vi "Set Velocity Setpoint.vi"(8 "error in (no error)":errorcluster, 10 "ccw velocity (rpm)":dbl, 11 "KUKA youBot gripper motor in":refnum<class "NI_Robotics_KUKA youBot Gripper Motor_EtherCAT.lvclass">) -> (0 "error out":errorcluster, 3 "KUKA youBot gripper motor out":refnum<class "NI_Robotics_KUKA youBot Gripper Motor_EtherCAT.lvclass">)   [LabVIEW 2017, in "NI_Robotics_KUKA youBot Host.lvlib" / "NI_Robotics_KUKA youBot Gripper Motor_EtherCAT.lvclass"]
uses:
  <vilib>/robotics/KUKA youBot/Motor/Gripper Motor EtherCAT/NI_Robotics_KUKA youBot Gripper Motor_EtherCAT.lvclass
  <vilib>/robotics/KUKA youBot/Motor/Gripper Motor EtherCAT/NI_Robotics_KUKA youBot Gripper Motor_EtherCAT.lvclass/NI_Robotics_KUKA youBot Gripper Motor_EtherCAT.ctl
  <vilib>/robotics/KUKA youBot/EtherCAT/EtherCAT Command.ctl
  <vilib>/robotics/KUKA youBot/EtherCAT/CmdCtrls/Param Cmd.ctl
  <vilib>/robotics/KUKA youBot/NI_Robotics_KUKA youBot Host.lvlib
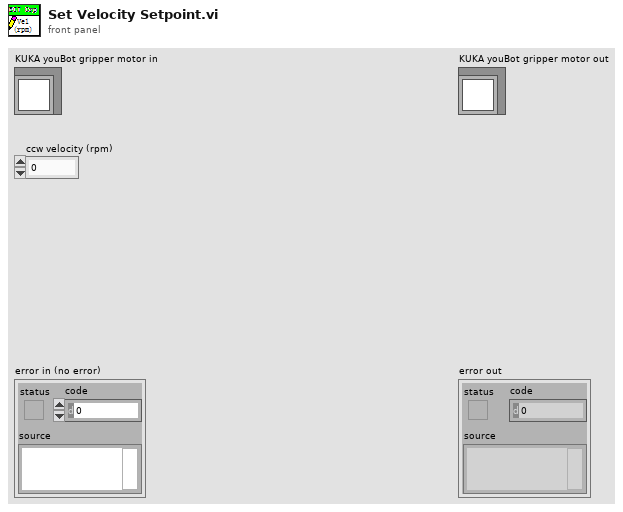
[diagram p1: front panel]
types:
  T1 = typedef "NI_Robotics_KUKA youBot Host.lvlib/EtherCAT Command.ctl" = cluster{"Module":u8, "Cmd":T2, "Type":u8, "Bank":u8, "Val":u32}
  T2 = typedef "NI_Robotics_KUKA youBot Host.lvlib/Param Cmd.ctl" = u8
  T3 = typedef "NI_Robotics_KUKA youBot Host.lvlib/Mater Handler.ctl" = i32
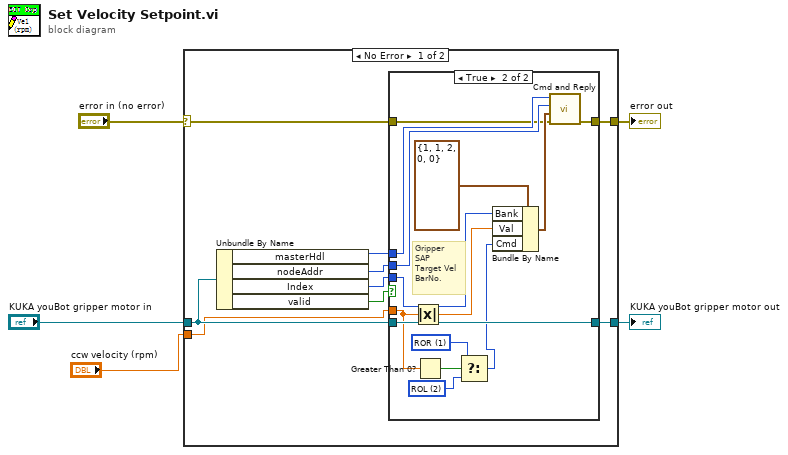
[diagram p0: block diagram]
diagram:
  n1 = case shown="No Error" "error in (no error)" {
    selector: "error in (no error)" -> [w8 w31]
    tunnel: "KUKA youBot gripper motor in" -> [w10 w32]
    tunnel: "ccw velocity (rpm)" -> [w9 _]
    tunnel: [w7 w32] -> w2
    tunnel: [w6 w31] -> w1
    frame No Error {
      n2 = Unbundle By Name(w10) -> ("masterHdl"=w14:T3, "nodeAddr"=w13:u16, "Index"=w12:i32, "valid"=w11:bool)
      n3 = case shown="True" w11 {
        tunnel: w8 -> [w15 w24]
        tunnel: w9 -> [_ w21]
        tunnel: w10 -> [w16 w23]
        tunnel: w14 -> [_ w30]
        tunnel: w13 -> [_ w29]
        tunnel: w12 -> [_ w27]
        tunnel: [w16 w23] -> w7
        tunnel: [w15 w25] -> w6
        frame False {
        }
        frame True {
          w18 = T2 2 items=["NONE", "ROR", "ROL", "MST", "MVP", "SAP", "GAP", "STAP", "RSAP"] ("Cmd")
          w19 = T2 1 items=["NONE", "ROR", "ROL", "MST", "MVP", "SAP", "GAP", "STAP", "RSAP"] ("Cmd")
          # "Gripper\nSAP\nTarget Vel\nBarNo."
          n4 = Absolute Value(x=w21) -> (abs(x)=w22:dbl)
          n5 = Greater Than 0?(x=w21) -> (x > 0?=w20:bool)
          n6 = Select(t=w19, s=w20, f=w18) -> (s? t:f=w17:T2)
          n7 = Bundle By Name(cluster=T1 {"Module"=1, "Cmd"=1, "Type"=2, "Bank"=0, "Val"=0} ("EtherCAT Command"), "Bank"=w27, "Val"=w22, "Cmd"=w17) -> (w26:T1)
          n8 = call <vilib>:"Cmd and Reply.vi"("error in (no error)"=w24, "EtherCAT command"=w26, "nodeAddr in"=w29, "masterHdl in"=w30) -> ("error out"=w25:errorcluster)  [unwired: 3 in, 4 out]
        }
      }
    }
    frame Error {
    }
  }
  "error out" <- w1
  "KUKA youBot gripper motor out" <- w2
